vi "ief_start_auto.vi"(0 "Tagprefix in":refnum<k21>, 1 "error in (no error)":errorcluster) -> (2 "Tagprefix out":refnum<k21>, 3 "PA Control State":u16, 4 "error out (no error)":errorcluster)   [LabVIEW 2015, in "IEF Werner.lvlib"]
doc: "The VI starts the automatic mode.\n\nPA Control State:\n000B hex, 11 dec - command executed without error"
uses:
  IEF Werner.lvlib
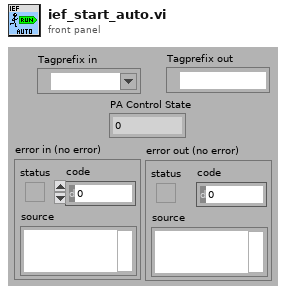
[diagram p1: front panel]
types:
  T1 = typedef "Semaphore RefNum" = refnum<k1>
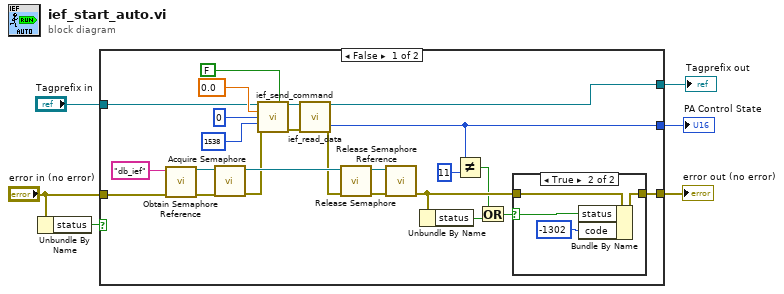
[diagram p0: block diagram]
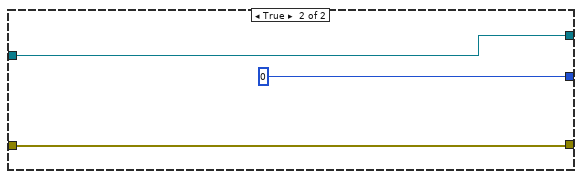
[diagram p3: hidden frame]
diagram:
  n1 = Unbundle By Name("error in (no error)") -> ("status"=w5:bool)
  n2 = case shown="False" w5 {
    tunnel: "error in (no error)" -> [w21 w38]
    tunnel: [w20 w38] -> w4
    tunnel: [w12 u8 0 ("PA Control state")] -> w3
    tunnel: "Tagprefix in" -> [w9 w37]
    tunnel: [w7 w37] -> w1
    frame False {
      n3 = call <vilib>:"Obtain Semaphore Reference.vi"("error in (no error)"=w21, "name (unnamed)"="db_ief") -> ("error out"=w28:errorcluster, "semaphore"=w29:T1)  [unwired: 3 in, 1 out]
      n4 = call <vilib>:"Acquire Semaphore.vi"("error in (no error)"=w28, "semaphore"=w29) -> ("error out"=w26:errorcluster, "semaphore out"=w27:T1)  [unwired: 3 in, 1 out]
      n5 = call "ief_send_command.vi"("Tagprefix in"=w9, "Command datum of type real"=FALSE, "Command datum"=sgl 0.0, "Command parameter"=u16 0, "Command code"=u16 1538, "error in (no error)"=w26) -> ("Tagprefix out"=w8:refnum<k21>, "error out (no error)"=w18:errorcluster)  [unwired: 4 in, 4 out]
      n6 = call "ief_read_data.vi"("Tagprefix in"=w8, "error in (no error)"=w18) -> ("Tagprefix out"=w7:refnum<k21>, "PA Control state"=w12:u8, "error out (no error)"=w17:errorcluster)  [unwired: 7 in, 4 out]
      n7 = call <vilib>:"Release Semaphore.vi"("error in (no error)"=w17, "semaphore"=w27) -> ("error out"=w25:errorcluster, "semaphore out"=w24:T1)  [unwired: 4 in]
      n8 = call <vilib>:"Release Semaphore Reference.vi"("error in (no error)"=w25, "semaphore"=w24) -> ("error out"=w19:errorcluster)  [unwired: 8 in, 1 out]
      n9 = Unbundle By Name(w19) -> ("status"=w13:bool)
      n10 = Not Equal?(x=w12, y=u16 11) -> (x != y?=w10:bool)
      n11 = Or(x=w10, y=w13) -> (x .or. y?=w14:bool)
      n12 = case shown="True" w14 {
        selector: w14 -> [_ w32]
        tunnel: [w31 w34] -> w20
        tunnel: w19 -> [w31 w35]
        frame False {
        }
        frame True {
          n13 = Bundle By Name(cluster=w35, "status"=w32, "code"=-1302) -> (w34:errorcluster)
        }
      }
    }
    frame True {
    }
  }
  "error out (no error)" <- w4
  "PA Control State" <- w3
  "Tagprefix out" <- w1
